vi "testStringArrayToStringWithBrackets.vi"(8 "error in (no error)":errorcluster) -> (0 "error out":errorcluster)   [LabVIEW 2018]
uses:
  <vilib>/addons/_JKI Toolkits/Caraya/classes/Assert/Assert Equal Value_Variant.vi
  <vilib>/addons/_JKI Toolkits/Caraya/classes/Test/Test.lvclass
  <vilib>/addons/_JKI Toolkits/Caraya/classes/Assert/Assert.lvclass
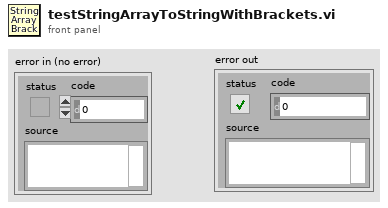
[diagram p1: front panel]
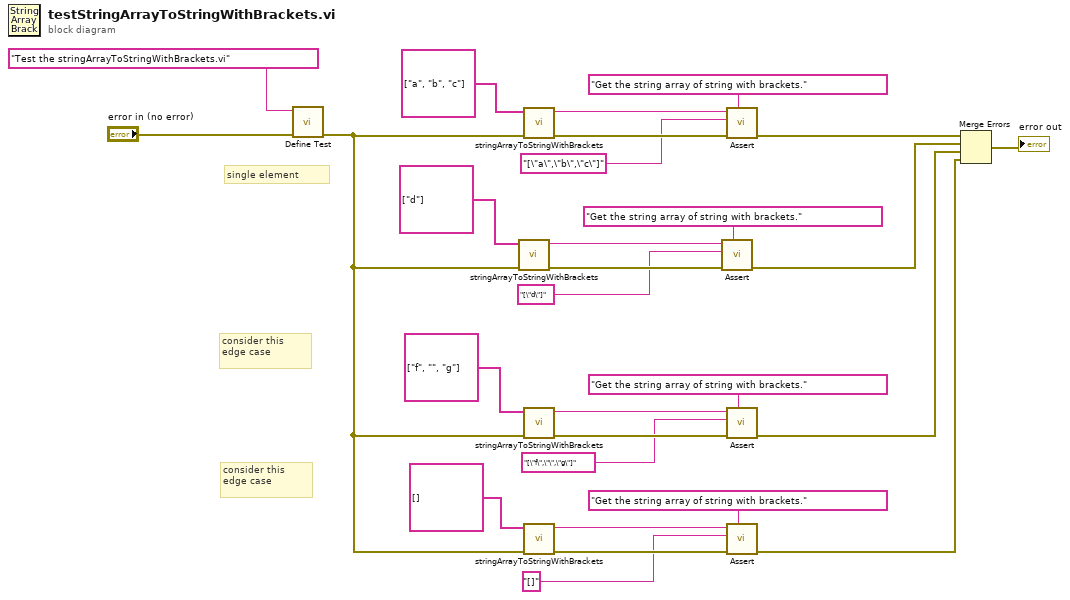
[diagram p0: block diagram]
diagram:
  # "single element"
  # "consider this\nedge case"
  # "consider this\nedge case"
  n1 = call <vilib>:"Define Test.vi"("error in (no error)"="error in (no error)", "Label (VI Title)"="Test the stringArrayToStringWithBrackets.vi") -> ("error out"=w1:errorcluster)  [unwired: 9 in]
  n2 = call "stringArrayToStringWithBrackets.vi"("error in (no error)"=w1, "value"=string[] ["d"]) -> ("error out"=w6:errorcluster, "String"=w7:string)  [unwired: 8 in]
  n3 = call "stringArrayToStringWithBrackets.vi"("error in (no error)"=w1, "value"=string[] ["a", "b", "c"]) -> ("error out"=w25:errorcluster, "String"=w26:string)  [unwired: 8 in]
  n4 = call "stringArrayToStringWithBrackets.vi"("error in (no error)"=w1, "value"=string[] ["f", "", "g"]) -> ("error out"=w22:errorcluster, "String"=w21:string)  [unwired: 8 in]
  n5 = call "stringArrayToStringWithBrackets.vi"("error in (no error)"=w1, "value"=string[] []) -> ("error out"=w19:errorcluster, "String"=w20:string)  [unwired: 8 in]
  n6 = call-poly <vilib>:"Assert.vi"("Label"="Get the string array of string with brackets.", "error in (no error)"=w6, "Y"="[\"d\"]" ("value"), "X"=w7) -> ("error out"=w2:errorcluster)  [unwired: 7 in]
  n7 = call-poly <vilib>:"Assert.vi"("Label"="Get the string array of string with brackets.", "error in (no error)"=w25, "Y"="[\"a\",\"b\",\"c\"]" ("value"), "X"=w26) -> ("error out"=w17:errorcluster)  [unwired: 7 in]
  n8 = call-poly <vilib>:"Assert.vi"("Label"="Get the string array of string with brackets.", "error in (no error)"=w22, "Y"="[\"f\",\"\",\"g\"]" ("value"), "X"=w21) -> ("error out"=w3:errorcluster)  [unwired: 7 in]
  n9 = call-poly <vilib>:"Assert.vi"("Label"="Get the string array of string with brackets.", "error in (no error)"=w19, "Y"="[]" ("value"), "X"=w20) -> ("error out"=w16:errorcluster)  [unwired: 7 in]
  n10 = Merge Errors(w17, w2, w3, w16) -> (→"error out":errorcluster)
